vi "SELECT_CHANEL.vi"(0 "VISA resource name":refnum<visa-resource-name>="GPIB0::1::INSTR", 1 "CH4":bool, 2 "CH3":bool, 3 "CH2":bool, 4 "CH1":bool) -> ()   [LabVIEW 2011]
panel:
  # "TDS 2014B"
  # "Select Channel"
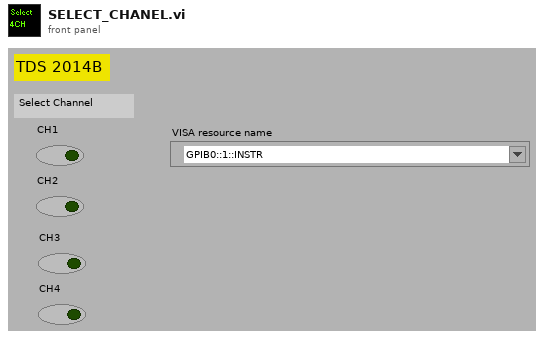
[diagram p1: front panel]
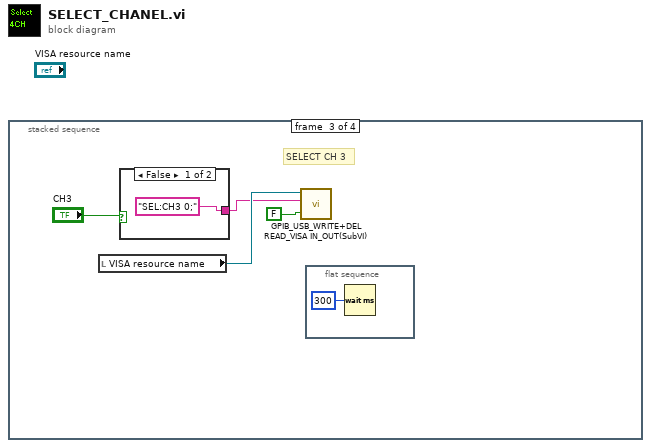
[diagram p0: block diagram]
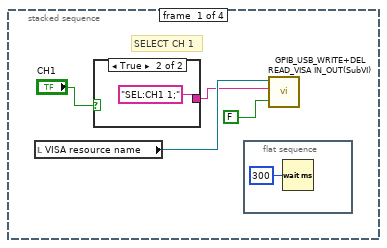
[diagram p2: hidden frame]
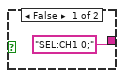
[diagram p3: hidden frame]
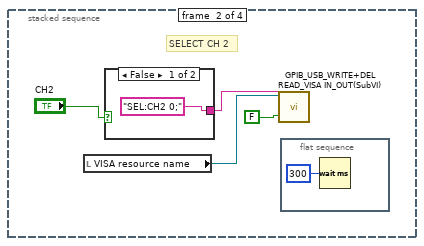
[diagram p4: hidden frame]
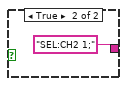
[diagram p5: hidden frame]
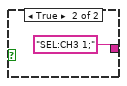
[diagram p6: hidden frame]
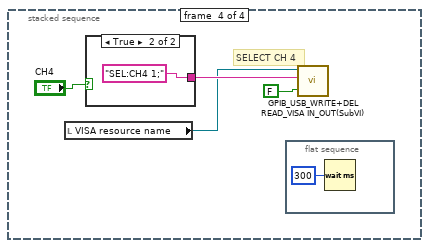
[diagram p7: hidden frame]
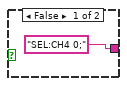
[diagram p8: hidden frame]
diagram:
  n1 = stacked-sequence {
    frame #0 {
      # "SELECT CH 1"
      n2 = local read "VISA resource name"() -> (w4:refnum<visa-resource-name>)
      n3 = case shown="True" "CH1" {
        tunnel: ["SEL:CH1 0;" "SEL:CH1 1;"] -> w3
        frame False {
        }
        frame True {
        }
      }
      n4 = flat-sequence {
        frame #0 {
          n5 = Wait (ms)(milliseconds to wait=u32 300) -> ()  [unwired: 1 out]
        }
      }
      n6 = call "GPIB_USB_WRITE+DEL READ_VISA IN_OUT(SubVI).vi"("VISA resource IN"=w4, "GPIB/USB WRITE"=w3, 4:FALSE ("READ GPIB")) -> ()  [unwired: 3 in, 3 out]
    }
    frame #1 {
      # "SELECT CH 2"
      n7 = local read "VISA resource name"() -> (w11:refnum<visa-resource-name>)
      n8 = case shown="False" "CH2" {
        tunnel: ["SEL:CH2 0;" "SEL:CH2 1;"] -> w10
        frame False {
        }
        frame True {
        }
      }
      n9 = call "GPIB_USB_WRITE+DEL READ_VISA IN_OUT(SubVI).vi"("VISA resource IN"=w11, "GPIB/USB WRITE"=w10, 4:FALSE ("READ GPIB")) -> ()  [unwired: 3 in, 3 out]
      n10 = flat-sequence {
        frame #0 {
          n11 = Wait (ms)(milliseconds to wait=u32 300) -> ()  [unwired: 1 out]
        }
      }
    }
    frame #2 {
      # "SELECT CH 3"
      n12 = local read "VISA resource name"() -> (w18:refnum<visa-resource-name>)
      n13 = case shown="False" "CH3" {
        tunnel: ["SEL:CH3 0;" "SEL:CH3 1;"] -> w17
        frame False {
        }
        frame True {
        }
      }
      n14 = call "GPIB_USB_WRITE+DEL READ_VISA IN_OUT(SubVI).vi"("VISA resource IN"=w18, "GPIB/USB WRITE"=w17, 4:FALSE ("READ GPIB")) -> ()  [unwired: 3 in, 3 out]
      n15 = flat-sequence {
        frame #0 {
          n16 = Wait (ms)(milliseconds to wait=u32 300) -> ()  [unwired: 1 out]
        }
      }
    }
    frame #3 {
      # "SELECT CH 4"
      n17 = local read "VISA resource name"() -> (w24:refnum<visa-resource-name>)
      n18 = case shown="True" "CH4" {
        tunnel: ["SEL:CH4 0;" "SEL:CH4 1;"] -> w25
        frame False {
        }
        frame True {
        }
      }
      n19 = flat-sequence {
        frame #0 {
          n20 = Wait (ms)(milliseconds to wait=u32 300) -> ()  [unwired: 1 out]
        }
      }
      n21 = call "GPIB_USB_WRITE+DEL READ_VISA IN_OUT(SubVI).vi"("VISA resource IN"=w24, "GPIB/USB WRITE"=w25, 4:FALSE ("READ GPIB")) -> ()  [unwired: 3 in, 3 out]
    }
  }
